vi "Get coord (SubVI).vi"(6 "Array":i32[](array[numeric]), 7 "Array 6":i32[](array[numeric]), 8 "Array 2":i32[](array[numeric]), 9 "Array 3":i32[](array[numeric]), 10 "Array 4":i32[](array[numeric]), 11 "Array 5":i32[](array[numeric])) -> (0 "String 2":string, 1 "String 3":string, 2 "String 4":string, 3 "String 5":string, 4 "String":string, 5 "String 6":string)   [LabVIEW 2015]
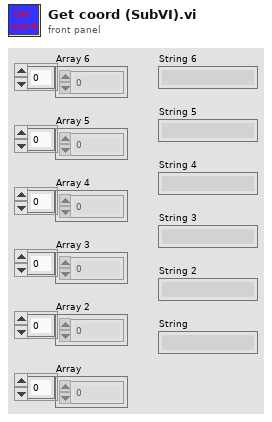
[diagram p1: front panel]
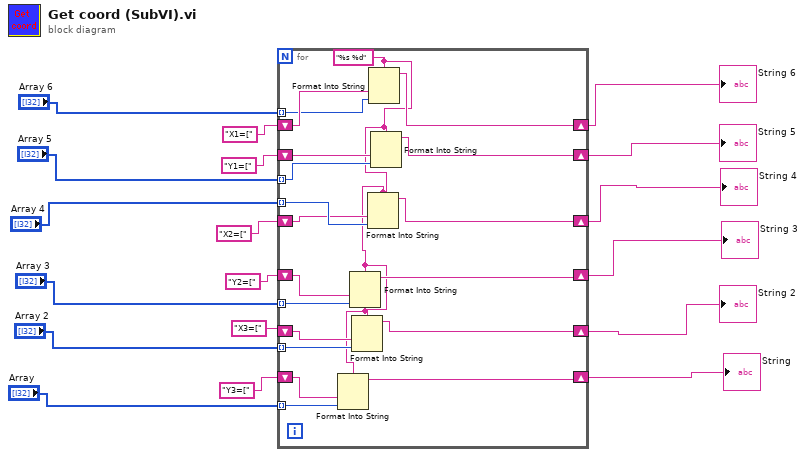
[diagram p0: block diagram]
diagram:
  n1 = for {
    shift-right: [w35] -> w8
    shift-left: "X1=[" -> [w37]
    tunnel: "Array 6" -> [w36] mode=indexing
    shift-right: [w32] -> w10
    shift-left: "Y1=[" -> [w34]
    tunnel: "Array 5" -> [w33] mode=indexing
    tunnel: "Array 4" -> [w31] mode=indexing
    shift-right: [w29] -> w12
    shift-left: "X2=[" -> [w30]
    shift-right: [w26] -> w14
    shift-left: "Y2=[" -> [w28]
    tunnel: "Array 3" -> [w27] mode=indexing
    shift-right: [w23] -> w17
    shift-left: "X3=[" -> [w25]
    shift-right: [w20] -> w18
    shift-left: "Y3=[" -> [w22]
    tunnel: "Array 2" -> [w24] mode=indexing
    tunnel: "Array" -> [w21] mode=indexing
    w19 = "%s %d" ("format string")
    n2 = Format Into String(format string=w19, w22, w21) -> (resulting string=w20:string)  [unwired: 2 in, 1 out]
    n3 = Format Into String(format string=w19, w28, w27) -> (resulting string=w26:string)  [unwired: 2 in, 1 out]
    n4 = Format Into String(format string=w19, w25, w24) -> (resulting string=w23:string)  [unwired: 2 in, 1 out]
    n5 = Format Into String(format string=w19, w30, w31) -> (resulting string=w29:string)  [unwired: 2 in, 1 out]
    n6 = Format Into String(format string=w19, w37, w36) -> (resulting string=w35:string)  [unwired: 2 in, 1 out]
    n7 = Format Into String(format string=w19, w34, w33) -> (resulting string=w32:string)  [unwired: 2 in, 1 out]
  }
  "String" <- w18
  "String 2" <- w17
  "String 3" <- w14
  "String 4" <- w12
  "String 5" <- w10
  "String 6" <- w8
